vi "GetVbreakStopTdmConfig.vi"(0 "storage refnum (file)":refnum<k20>, 1 "error in":errorcluster) -> (2 "storage refnum (file) out":refnum<k20>, 3 "output cluster":T1, 4 "error out":errorcluster)   [LabVIEW 2014]
uses:
  VBreakStopCondition.ctl
  <vilib>/Platform/storage/lvStorage.llb/_queryPropPoly.vi
  <vilib>/Platform/storage/lvStorage.llb/_queryPropString.vi
  <vilib>/Platform/storage/lvStorage.llb/_queryGenericObjects.vi
  <vilib>/Platform/storage/lvStorage.llb/_loadAllDdt.vi
  <vilib>/Platform/storage/lvStorage.llb/xStorage/xStorageSupp/ErrorOut.vi
  <vilib>/Platform/storage/lvStorage.llb/xStorage/Read Data/Read Data.xnode
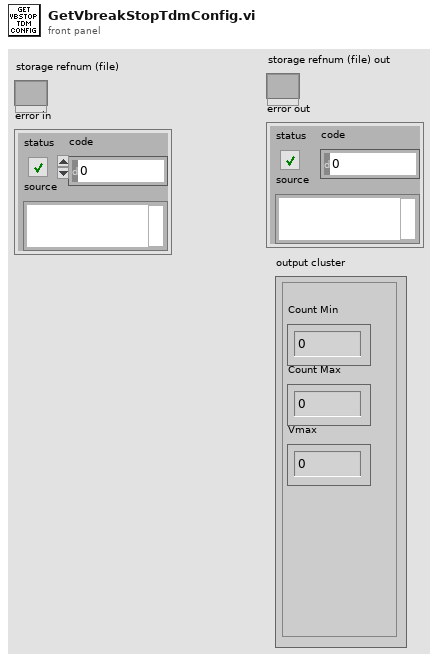
[diagram p1: front panel]
types:
  T1 = typedef "VBreakStopCondition.ctl" = cluster{"Count Min":dbl, "Count Max":dbl, "Vmax":dbl}
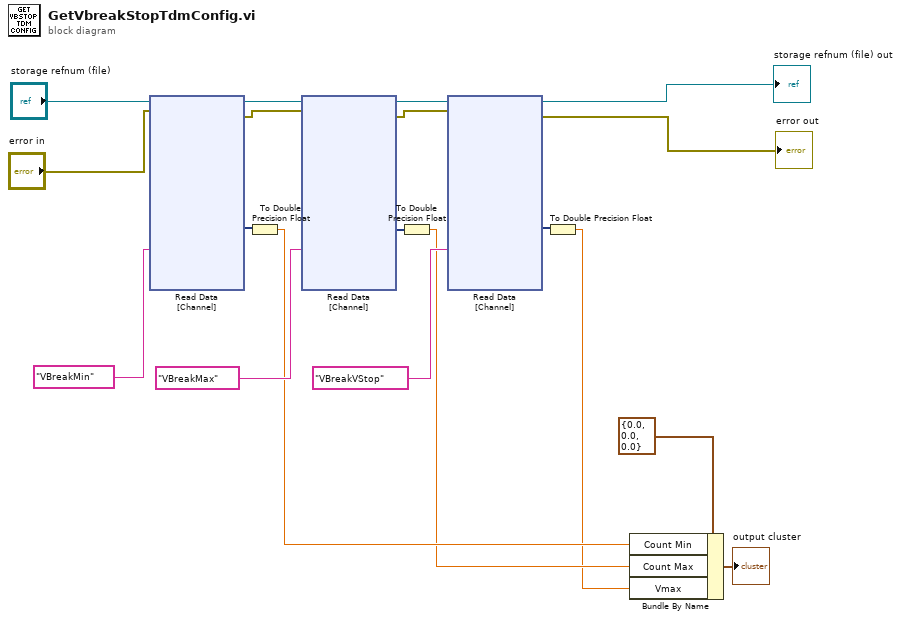
[diagram p0: block diagram]
diagram:
  n1 = xnode "Read Data\n[Channel]"("Name"="VBreakMin", "storage refnum (file)"="storage refnum (file)", "error in"="error in") -> ("Signal"=w19:dynamicdata, "storage refnum (file) out"=w16:refnum<k20>, "error out"=w14:errorcluster)  [unwired: 3 in, 1 out]
  n2 = To Double Precision Float(number=w19) -> (double precision float=w7:dbl)
  n3 = xnode "Read Data\n[Channel]"("Name"="VBreakMax", "storage refnum (file)"=w16, "error in"=w14) -> ("Signal"=w18:dynamicdata, "storage refnum (file) out"=w15:refnum<k20>, "error out"=w13:errorcluster)  [unwired: 3 in, 1 out]
  n4 = To Double Precision Float(number=w18) -> (double precision float=w6:dbl)
  n5 = xnode "Read Data\n[Channel]"("Name"="VBreakVStop", "storage refnum (file)"=w15, "error in"=w13) -> ("Signal"=w17:dynamicdata, "storage refnum (file) out"=→"storage refnum (file) out":refnum<k20>, "error out"=→"error out":errorcluster)  [unwired: 3 in, 1 out]
  n6 = To Double Precision Float(number=w17) -> (double precision float=w5:dbl)
  n7 = Bundle By Name(cluster=T1 {"Count Min"=0.0, "Count Max"=0.0, "Vmax"=0.0} ("Condition d'arret"), "Count Min"=w7, "Count Max"=w6, "Vmax"=w5) -> (→"output cluster":T1)
